vi "read_In0.vi"() -> (0 "INMFC1":dbl, 1 "Remote":bool, 2 "Run":bool, 3 "Bubbler In":bool, 4 "Active":bool)   [LabVIEW 2011]
uses:
  low_level_proc/globals.vi
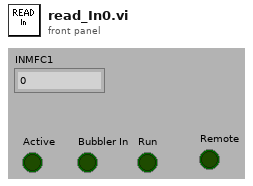
[diagram p1: front panel]
types:
  T1 = typedef "relaySpec.ctl" = cluster{"Card Index":u16, "Relay Index":u16}
  T2 = cluster{"P Gas":cluster{"Remote":T1, "Active":T1, "Gas In":T1, "H2 Flush":T1, "Run":T1}, "Ga bubbler":cluster{"Remote":T1, "Active":T1, "Bubbler In":T1, "Run":T1, "H2 Dilute":T1}, "In bubbler":cluster{"Remote":T1, "Active":T1, "Bubbler In":T1, "Run":T1}, "Al bubbler":cluster{"Remote":T1, "Active":T1, "Bubbler In":T1, "Run":T1}, "As Gas":cluster{"Remote":T1, "Active":T1, "Gas In":T1, "H2 Flush":T1, "Run":T1}, "H2/N2":cluster{"Remote":T1, "H2 On":T1, "N2 On":T1, "Output":T1}}
  T3 = cluster{"Remote":T1, "Active":T1, "Bubbler In":T1, "Run":T1}
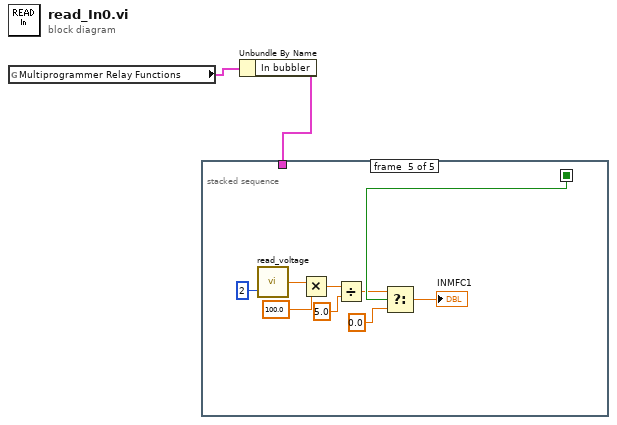
[diagram p0: block diagram]
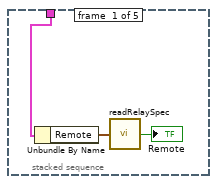
[diagram p2: hidden frame]
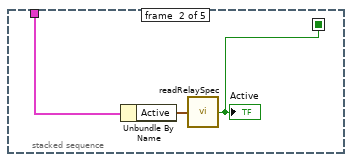
[diagram p3: hidden frame]
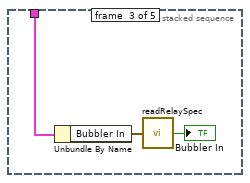
[diagram p4: hidden frame]
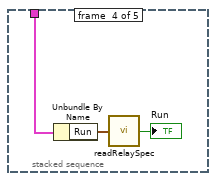
[diagram p5: hidden frame]
diagram:
  n1 = global read "globals.vi" "Multiprogrammer Relay Functions"() -> (w2:T2)
  n2 = Unbundle By Name(w2) -> ("In bubbler"=w1:T3)
  n3 = stacked-sequence {
    seq-local: [_ w8 _ _ _] -> [_ _ _ _ w18]
    tunnel: w1 -> [w4 w7 w10 w13 _]
    frame #0 {
      n4 = Unbundle By Name(w4) -> ("Remote"=w3:T1)
      n5 = call "readRelaySpec.vi"("RelaySpec"=w3) -> ("Relay Status"=→"Remote":bool)
    }
    frame #1 {
      n6 = Unbundle By Name(w7) -> ("Active"=w6:T1)
      n7 = call "readRelaySpec.vi"("RelaySpec"=w6) -> ("Relay Status"=w8:bool)
      "Active" <- w8
    }
    frame #2 {
      n8 = Unbundle By Name(w10) -> ("Bubbler In"=w9:T1)
      n9 = call "readRelaySpec.vi"("RelaySpec"=w9) -> ("Relay Status"=→"Bubbler In":bool)
    }
    frame #3 {
      n10 = Unbundle By Name(w13) -> ("Run"=w12:T1)
      n11 = call "readRelaySpec.vi"("RelaySpec"=w12) -> ("Relay Status"=→"Run":bool)
    }
    frame #4 {
      n12 = call "read_voltage.vi"("Channel"=2) -> ("Voltage"=w22:dbl)  [unwired: 1 in]
      n13 = Multiply(x=w22, y=100.0) -> (x*y=w20:dbl)
      n14 = Divide(x=w20, y=5.0) -> (x/y=w17:dbl)
      n15 = Select(t=w17, s=w18, f=0.0) -> (s? t:f=→"INMFC1":dbl)
    }
  }
